vi "SubPV.vi"(0 "v_DC(k-1)":fxp<+,28,8>, 1 "1-D_P":fxp<+,20,0>, 3 "v_pv(k-1)":fxp<+,26,6>, 4 "i_pv(k-1)":fxp<+,24,4>, 6 "i_L_P(k-1)":fxp<+/-,27,7>) -> (7 "i_P":fxp<+/-,25,5>, 15 "i_L_P(k)":fxp<+/-,27,7>, 18 "v_pv(k)":fxp<+,26,6>)   [LabVIEW 2015]
uses:
  <vilib>/rvi/FXPMathLib/FxpMul/XNode/nifxpmath_Multiplier.xnode
  <vilib>/rvi/FXPMathLib/FxpAdd/XNode/nifxpmath_Add.xnode
  <vilib>/rvi/FXPMathLib/FxpSub/XNode/nifxpmath_Sub.xnode
  <vilib>/rvi/FXPMathLib/sim/FxpSim.dll
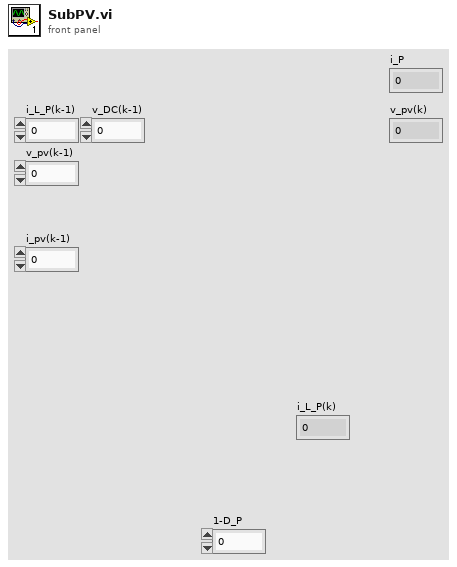
[diagram p1: front panel]
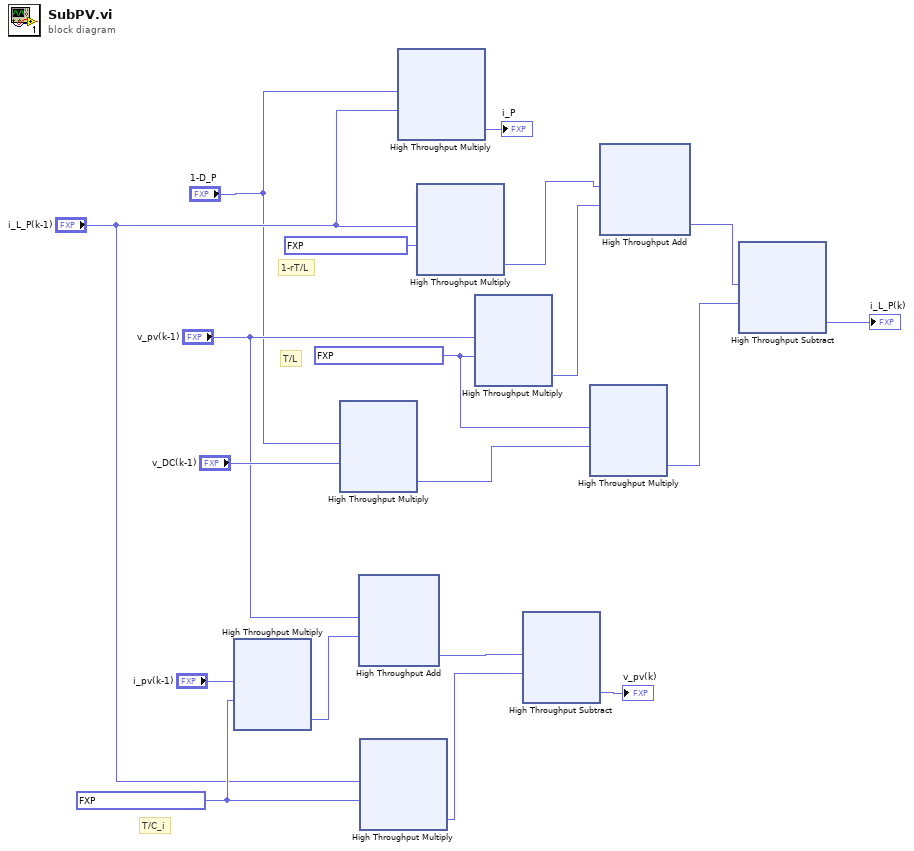
[diagram p0: block diagram]
diagram:
  w7 = fxp<+,20,0> 0.08484840393066406 ("y")
  w3 = fxp<+,20,0> 0.2545452117919922 ("y")
  # "T/C_i"
  # "T/L"
  # "1-rT/L"
  n1 = xnode ("High Throughput Multiply")("x"="i_pv(k-1)", "y"=w7) -> ("x*y"=w10:fxp<+,44,4>)
  n2 = xnode ("High Throughput Multiply")("x"="1-D_P", "y"="v_DC(k-1)") -> ("x*y"=w2:fxp<+,48,8>)
  n3 = xnode ("High Throughput Add")("x"="v_pv(k-1)", "y"=w10) -> ("x+y"=w12:fxp<+,47,7>)
  n4 = xnode ("High Throughput Multiply")("x"="i_L_P(k-1)", "y"=w7) -> ("x*y"=w8:fxp<+/-,47,7>)
  n5 = xnode ("High Throughput Multiply")("x"="1-D_P", "y"="i_L_P(k-1)") -> ("x*y"=→"i_P":fxp<+/-,25,5>)
  n6 = xnode ("High Throughput Multiply")("x"="i_L_P(k-1)", "y"=fxp<+,20,0> 0.8981819152832031) -> ("x*y"=w18:fxp<+/-,47,7>)
  n7 = xnode ("High Throughput Multiply")("x"="v_pv(k-1)", "y"=w3) -> ("x*y"=w17:fxp<+,46,6>)
  n8 = xnode "High Throughput Subtract"("x"=w12, "y"=w8) -> ("x-y"=→"v_pv(k)":fxp<+,26,6>)
  n9 = xnode ("High Throughput Multiply")("x"=w3, "y"=w2) -> ("x*y"=w16:fxp<+,64,8>)
  n10 = xnode ("High Throughput Add")("x"=w18, "y"=w17) -> ("x+y"=w19:fxp<+/-,48,8>)
  n11 = xnode "High Throughput Subtract"("x"=w19, "y"=w16) -> ("x-y"=→"i_L_P(k)":fxp<+/-,27,7>)
